vi "WPI_Gyro_ADXRS453_SPIToBitArray.vi"(11 "SPI Byte Array (MSB first)":u8[](array[numeric])) -> (3 "32-bit Boolean array":bool[](array[boolean]))   [LabVIEW 2017]
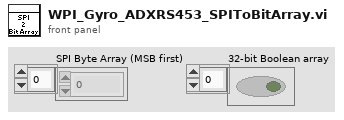
[diagram p1: front panel]
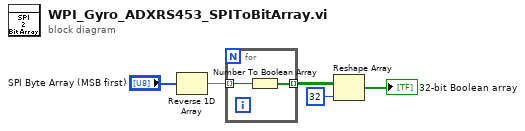
[diagram p0: block diagram]
diagram:
  n1 = Reverse 1D Array(array="SPI Byte Array (MSB first)") -> (reversed array=w2:u8[])
  n2 = for {
    tunnel: w2 -> [w7] mode=indexing
    tunnel: [w6] -> w4 mode=indexing
    n3 = Number To Boolean Array(number=w7) -> (Boolean array=w6:bool[])
  }
  n4 = Reshape Array(w4, 32 ("dimension size")) -> (→"32-bit Boolean array":bool[])
